vi "Get Timestamp Cushion.vi"(11 "DoubleTimestampRepresentation":dbl) -> (3 "TimestampCushion":dbl)   [LabVIEW 2016, in "M1M3SupportEUI_Views.lvlib"]
uses:
  M1M3SupportEUI_Views.lvlib
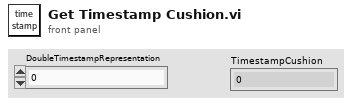
[diagram p1: front panel]
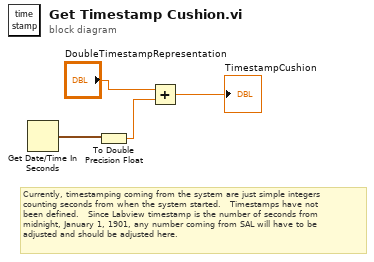
[diagram p0: block diagram]
diagram:
  # "Currently, timestamping coming from the system are just simple integers\ncounting seconds from when the system started.   Timestamps have not \nbeen defined.   Since Labview timestamp is the number of seconds from \nmidnight, January 1, 1901, any number coming from SAL will have to be \nadjusted and should be adjusted here."
  n1 = Get Date/Time In Seconds() -> (seconds since 1Jan1904=w4:timestamp)
  n2 = To Double Precision Float(number=w4) -> (double precision float=w2:dbl)
  n3 = Add(x="DoubleTimestampRepresentation", y=w2) -> (x+y=→"TimestampCushion":dbl)
